vi "数据主动和反控发送.vi"   [LabVIEW 2016, in "数据传输系统.lvlib"]
types:
  T1 = cluster{"CODMn":bool, "CODCr":bool, "DO":bool, "铜":bool, "PH":bool, "氨氮":bool, "比电导率":bool, "水温":bool, "盐度(海水)":bool, "浊度":bool, "总氮":bool, "总磷":bool, "叶绿素a":bool, "藻密度":bool, "水位":bool, "流速":bool, "瞬时流量":bool, "累积流量":bool}
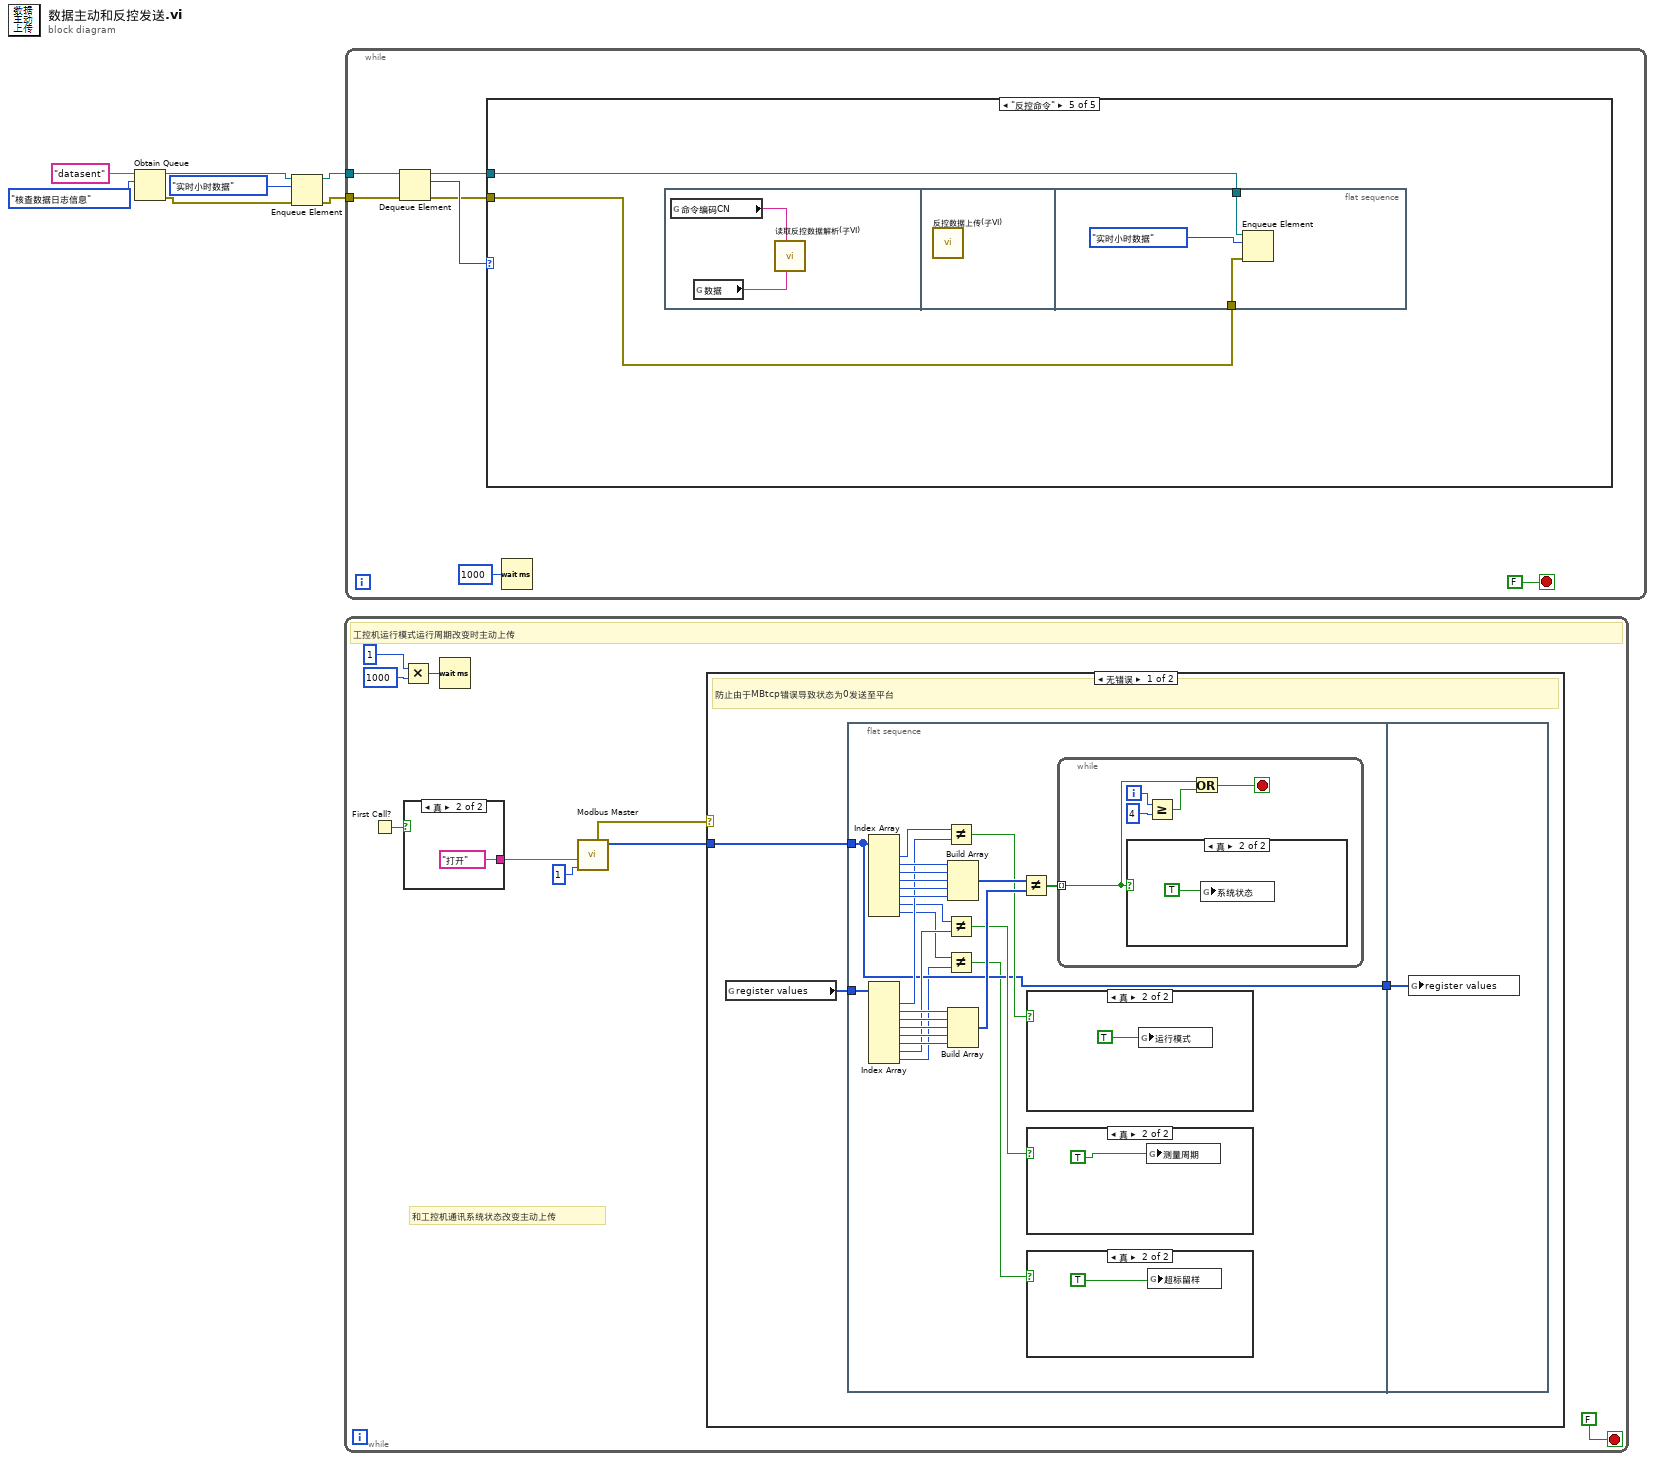
[diagram p0: block diagram]
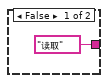
[diagram p7: hidden frame]
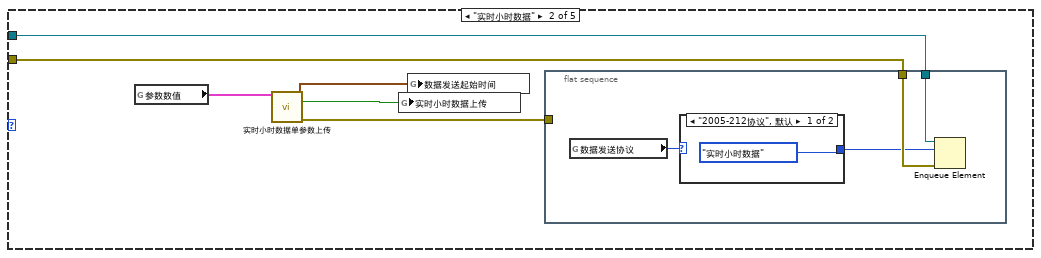
[diagram p9: hidden frame]
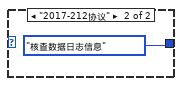
[diagram p10: hidden frame]
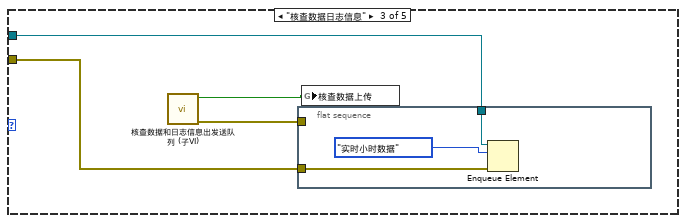
[diagram p11: hidden frame]
diagram:
  n1 = Obtain Queue(name (unnamed)="datasent" ("名称（未命名）"), element data type=enum16{"实时小时数据", "核查数据日志信息", "其他信息", "反控命令"}."核查数据日志信息") -> (queue out=w4:refnum<queue>, error out=w1:errorcluster)  [unwired: 3 in, 1 out]
  n2 = Enqueue Element(queue=w4, element=enum16{"实时小时数据", "核查数据日志信息", "其他信息", "反控命令"}."实时小时数据", error in (no error)=w1) -> (queue out=w3:refnum<queue>, error out=w2:errorcluster)  [unwired: 1 in, 1 out]
  n3 = while {
    stop <- FALSE stop-if-true
    # "和工控机通讯系统状态改变主动上传"
    # "工控机运行模式运行周期改变时主动上传"
    n4 = First Call?() -> (First Call?: T/F=w8:bool)
    n5 = Multiply(x=u32 1, y=u32 1000 ("等待时间（毫秒）")) -> (x*y=w15:u32)
    n6 = case shown="真" w8 {
      tunnel: ["读取" ("读取写入选择") "打开" ("读取写入选择")] -> w12
      frame False {
      }
      frame True {
      }
    }
    n7 = Wait (ms)(milliseconds to wait=w15) -> ()  [unwired: 1 out]
    n8 = call "Modbus Master.vi"("Unit ID"=u8 1, "读取写入选择"=w12) -> ("register values"=w10:u16[], "error out"=w9:errorcluster)  [unwired: 8 in]
    n9 = case shown="无错误" w9 {
      tunnel: w10 -> [w18 _]
      frame No Error {
        # "防止由于MBtcp错误导致状态为0发送至平台"
        n10 = global read "全局1.vi" "register values"() -> (w17:u16[])
        n11 = flat-sequence {
          tunnel: w18 -> [w23]
          tunnel: w17 -> [w43]
          tunnel: [w23] -> w19
          tunnel: w19 -> [w53]
          frame #0 {
            n12 = Index Array(array=w23) -> (element #1=w30:u16, element #2=w42:u16, element #3=w41:u16, element #4=w40:u16, element #5=w39:u16, element #6=w38:u16, element #7=w28:u16, element #8=w22:u16)  [unwired: 8 in]
            n13 = Index Array(array=w43) -> (element #1=w29:u16, element #2=w37:u16, element #3=w36:u16, element #4=w35:u16, element #5=w34:u16, element #6=w33:u16, element #7=w27:u16, element #8=w21:u16)  [unwired: 8 in]
            n14 = Not Equal?(x=w30, y=w29) -> (x != y?=w25:bool)
            n15 = Not Equal?(x=w28, y=w27) -> (x != y?=w26:bool)
            n16 = Not Equal?(x=w22, y=w21) -> (x != y?=w20:bool)
            n17 = Build Array(w42, w41, w40, w39, w38) -> (w32:u16[])
            n18 = Build Array(w37, w36, w35, w34, w33) -> (w31:u16[])
            n19 = Not Equal?(x=w32, y=w31) -> (x != y?=w24:bool[])
            n20 = case shown="真" w25 {
              frame False {
              }
              frame True {
                n21 = global write "全局1.vi" "运行模式"(TRUE) -> ()
              }
            }
            n22 = case shown="真" w26 {
              frame False {
              }
              frame True {
                n23 = global write "全局1.vi" "测量周期"(TRUE ("系统状态改变")) -> ()
              }
            }
            n24 = case shown="真" w20 {
              frame False {
              }
              frame True {
                n25 = global write "全局1.vi" "超标留样"(TRUE ("系统状态改变")) -> ()
              }
            }
            n26 = while {
              tunnel: w24 -> [w47] mode=indexing
              i -> [w49]
              stop <- w45 stop-if-true
              n27 = case shown="真" w47 {
                frame False {
                }
                frame True {
                  n28 = global write "全局1.vi" "系统状态"(TRUE ("系统状态改变")) -> ()
                }
              }
              n29 = Greater Or Equal?(x=w49, y=4) -> (x >= y?=w46:bool)
              n30 = Or(x=w47, y=w46) -> (x .or. y?=w45:bool)
            }
          }
          frame #1 {
            n31 = global write "全局1.vi" "register values"(w53) -> ()
          }
        }
      }
      frame Error {
      }
    }
  }
  n32 = while {
    tunnel: w3 -> [w60]
    tunnel: w2 -> [w59]
    stop <- FALSE stop-if-true
    n33 = Dequeue Element(queue=w60, error in (no error)=w59) -> (queue out=w57:refnum<queue>, element=w58:enum16{"实时小时数据", "核查数据日志信息", "其他信息", "反控命令"}, error out=w56:errorcluster)  [unwired: 1 in, 1 out]
    n34 = case shown="\"反控命令\"" w58 {
      tunnel: w57 -> [_ w66 w77 _ w83]
      tunnel: w56 -> [_ w65 w76 _ w82]
      frame Default {
      }
      frame "实时小时数据" {
        n35 = global read "全局1.vi" "参数数值"() -> (w68:T1)
        n36 = call "实时小时数据单参数上传.vi"("参数数值"=w68) -> ("数据发送起始时间"=w63:timestamp, "实时小时数据上传"=w64:bool, "error out"=w67:errorcluster)  [unwired: 12 in]
        n37 = global write "全局1.vi" "实时小时数据上传"(w64) -> ()
        n38 = global write "全局1.vi" "数据发送起始时间"(w63) -> ()
        n39 = flat-sequence {
          tunnel: w67 -> [_]
          tunnel: w66 -> [w71]
          tunnel: w65 -> [w70]
          frame #0 {
            n40 = global read "断电保存全局.vi" "数据发送协议"() -> (w72:enum16{"2005-212协议", "2017-212协议"})
            n41 = case shown="\"2005-212协议\", 默认" w72 {
              tunnel: [enum16{"实时小时数据", "核查数据日志信息", "其他信息", "反控命令"}."实时小时数据" enum16{"实时小时数据", "核查数据日志信息", "其他信息", "反控命令"}."核查数据日志信息"] -> w69
              frame "2005-212协议", Default {
              }
              frame "2017-212协议" {
              }
            }
            n42 = Enqueue Element(queue=w71, element=w69, error in (no error)=w70) -> ()  [unwired: 1 in, 3 out]
          }
        }
      }
      frame "核查数据日志信息" {
        n43 = call "核查数据和日志信息出发送队列 (子VI).vi"() -> ("错误输出"=w78:errorcluster, "核查数据上传"=w75:bool)  [unwired: 10 in]
        n44 = flat-sequence {
          tunnel: w78 -> [_]
          tunnel: w77 -> [w81]
          tunnel: w76 -> [w80]
          frame #0 {
            n45 = Enqueue Element(queue=w81, element=enum16{"实时小时数据", "核查数据日志信息", "其他信息", "反控命令"}."实时小时数据", error in (no error)=w80) -> ()  [unwired: 1 in, 3 out]
          }
        }
        n46 = global write "全局1.vi" "核查数据上传"(w75) -> ()
      }
      frame "其他信息" {
      }
      frame "反控命令" {
        n47 = flat-sequence {
          tunnel: w83 -> [w88]
          tunnel: w82 -> [w86]
          frame #0 {
            n48 = global read "全局1.vi" "命令编码CN"() -> (w85:string)
            n49 = global read "全局1.vi" "数据"() -> (w84:string)
            n50 = call "读取反控数据解析(子VI).vi"("数据"=w84, "命令编码CN"=w85) -> ()  [unwired: 8 in, 2 out]
          }
          frame #1 {
            n51 = call "反控数据上传(子VI).vi"() -> ()  [unwired: 12 in]
          }
          frame #2 {
            n52 = Enqueue Element(queue=w88, element=enum16{"实时小时数据", "核查数据日志信息", "其他信息", "反控命令"}."实时小时数据", error in (no error)=w86) -> ()  [unwired: 1 in, 3 out]
          }
        }
      }
    }
    n53 = Wait (ms)(milliseconds to wait=u32 1000 ("等待时间（毫秒）")) -> ()  [unwired: 1 out]
  }
